vi "Acq&Graph Voltage-Int Clk demo.vi"() -> ()   [LabVIEW 2010]
doc: "I. Description:\nThis example demonstrates how to acquire a finite amount of data (waveform) using the DAQ device's internal clock.\n\nII. Instructions for Running:\n1. Select the physical channel to correspond to where your signal is input on the DAQ device.\n2. Enter the minimum and maximum voltages.\nNote: For better accuracy try to match the input range to the expected voltage level of the measured signal.\n3. Select the number of samples to acquire.\n4. Set the rate of the acquisition\nNote: The rate should be AT LEAST twice as fast as the maximum frequency component of the signal being acquired.\n\nIII. Block Diagram Steps:\n1. Create an analog input voltage channel.\n2. Set the rate for the sample clock. Additionally, define the sample mode to be finite and set the number of samples to be acquired per channel.\n3. Call the Start VI to start the acquisition.\n4. Use the Read VI to measure multiple samples from N Channels on the device. Set a timeout so an error is returned if the samples are not returned in the specified time limit\n5. Call the Clear Task VI to clear the Task.\n6. Use the popup dialog box to display an error if any.\n \nIV. I/O Connections Overview:\nMake sure your signal input terminal matches the Physical Channel I/O Control. For further connection information, refer to your hardware reference manual."
uses:
  <vilib>/Utility/error.llb/DialogType.ctl
  <vilib>/DAQmx/read.llb/DAQmx Read (Analog 1D Wfm NChan NSamp).vi
  <vilib>/DAQmx/configure/timing.llb/DAQmx Timing (Sample Clock).vi
  <vilib>/DAQmx/create/channels.llb/DAQmx Create Channel (AI-Voltage-Basic).vi
  Program Files/National Instruments/LabVIEW 2010/resource/objmgr/daqmx.rc
panel:
  in  "groups":T1(array[cluster]) {"Maximum Value" format="%0.2f"}
  in  "millisecond multiple":u32
  out "data":waveform(dbl)[](array[waveform])
  in  "stop":bool
  in  "Rate":dbl=10000.0 caption="Sample Rate (Hz)" format="%0.2f"
  out "Measurement":waveform(dbl)[](graph)
  # "For instructions, select Help>>Show Context Help"
  # "Channel Parameters"
  # "Timing Parameters"
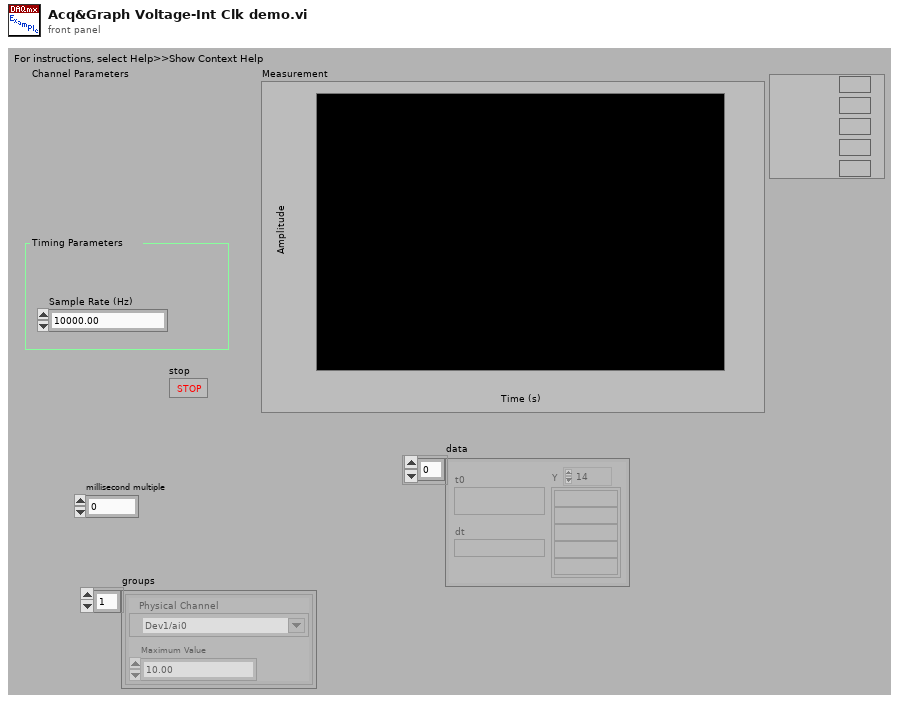
[diagram p1: front panel]
types:
  T1 = cluster{"Physical Channel":tag, "Maximum Value":dbl}[]
  T2 = typedef "DialogType.ctl" = u16
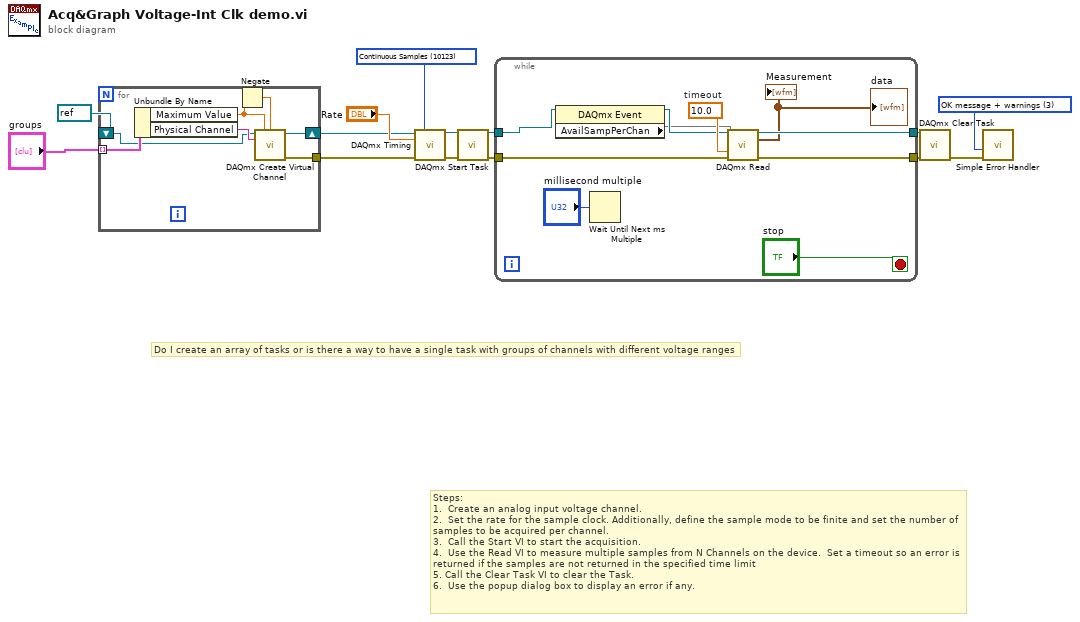
[diagram p0: block diagram]
diagram:
  w4 = T2 3 items=["no dialog", "OK message", "continue or stop message", "OK message + warnings", "continue/stop + warnings"] ("type of dialog (OK msg:1)")
  w8 = 10123 items=["Finite Samples"=10178, "Continuous Samples"=10123] ("sample mode")
  # "Do I create an array of tasks or is there a way to have a single task with groups of channels with different voltage ranges"
  # "Steps: \n1.  Create an analog input voltage channel.\n2.  Set the rate for the sample clock. Additionally, define the sample mode to be finite and set the number of samples to be acquired per channel.\n3.  Call the Start VI to start the acquisition.\n4.  Use the Read VI to measure multiple samples from N Channels on the device.  Set a timeout so an error is returned if the samples are not returned in the specified time limit\n5. Call the Clear Task VI to clear the Task.\n6.  Use the popup dialog box to display an error if any."
  n1 = for {
    tunnel: [w21] -> w14
    tunnel: "groups" -> [w19] mode=indexing
    shift-right: [w20] -> w3
    shift-left: refnum<k21> refnum ("task out") -> [w15]
    n2 = Unbundle By Name(w19) -> ("Maximum Value"=w18:dbl, "Physical Channel"=w16:tag)
    n3 = Negate(x=w18) -> (-x=w17:dbl)
    n4 = call-poly <vilib>:"DAQmx Create Virtual Channel.vi"("task in"=w15, "maximum value"=w18, "minimum value"=w17, "physical channels"=w16) -> ("task out"=w20:refnum<k21>, "error out"=w21:errorcluster)  [unwired: 10 in]
  }
  n5 = call-poly <vilib>:"DAQmx Timing.vi"("task/channels in"=w3, "sample mode"=w8, "rate"="Rate", "error in"=w14) -> ("task out"=w7:refnum<k21>, "error out"=w6:errorcluster)  [unwired: 10 in]
  n6 = call <vilib>:"DAQmx Start Task.vi"("task/channels in"=w7, "error in"=w6) -> ("task out"=w10:refnum<k21>, "error out"=w13:errorcluster)  [unwired: 12 in]
  n7 = while {
    tunnel: w13 -> [w31]
    tunnel: w10 -> [w25]
    tunnel: [w30] -> w9
    tunnel: [w28] -> w5
    stop <- "stop" stop-if-true
    w27 = 10.0  # timeout
    n8 = property class="DAQmx Event"(reference=w25) -> (reference out=w24:refnum<k21>, "AvailSampPerChan"=w23)  [unwired: 1 in, 1 out]
    n9 = Wait Until Next ms Multiple(millisecond multiple="millisecond multiple") -> ()  [unwired: 1 out]
    n10 = call-poly <vilib>:"DAQmx Read.vi"("task/channels in"=w24, "number of samples per channel"=w23, "timeout"=w27, "error in"=w31) -> ("task out"=w30:refnum<k21>, "data"=→"Measurement" →"data":waveform(dbl)[], "error out"=w28:errorcluster)  [unwired: 9 in]
  }
  n11 = call <vilib>:"DAQmx Clear Task.vi"("task in"=w9, "error in"=w5) -> ("error out"=w12:errorcluster)  [unwired: 13 in]
  n12 = call <vilib>:"Simple Error Handler.vi"("type of dialog (OK msg:1)"=w4, "error in (no error)"=w12) -> ()  [unwired: 3 in, 5 out]
